vi "SET_SAMPLINGRATE_DIVIDER_n.vi"(2 "execute":bool, 5 "ulValue":u32, 11 "error in (no error)":errorcluster) -> (4 "function return":string, 15 "error out":errorcluster)   [LabVIEW 2017, in "ZBOX_IS.lvlib"]
uses:
  ZBOX_IS.lvlib
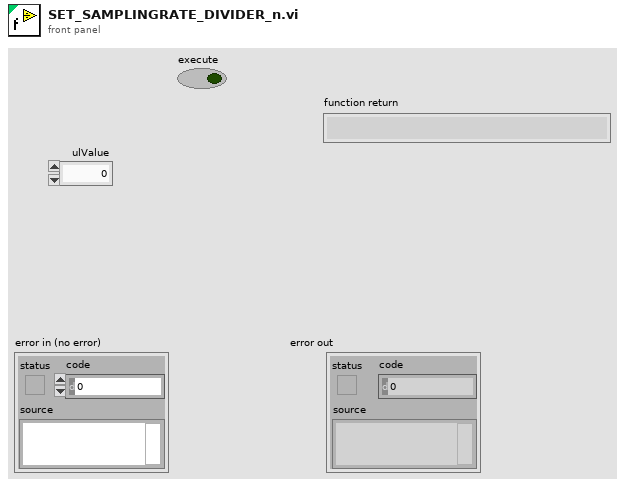
[diagram p1: front panel]
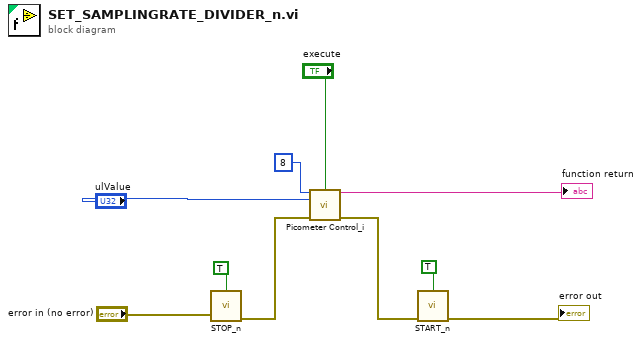
[diagram p0: block diagram]
diagram:
  n1 = call "STOP_n.vi"("execute"=TRUE, "error in (no error)"="error in (no error)") -> ("error out"=w5:errorcluster)  [unwired: 12 in, 1 out]
  n2 = call "Picometer Control_i.vi"("Cmd"=u8 8, "execute"="execute", "ulValue"="ulValue", "error in (no error)"=w5) -> ("function return"=→"function return":string, "error out"=w4:errorcluster)  [unwired: 7 in, 3 out]
  n3 = call "START_n.vi"("execute"=TRUE, "error in (no error)"=w4) -> ("error out"=→"error out":errorcluster)  [unwired: 12 in, 1 out]
